vi "ExecuteState.vi"(0 "StateIn":T7 {"ILoad" format="%_6g"; "Fault Registers" format="%016x"; "VLoad" format="%_6g"; "VDCLink" format="%_6g"; "Detected Frequency" format="%1_6g"}, 1 "Interfaces":T2, 7 "methods":T1, 9 "params":refnum<class "JSON Null.lvclass">, 11 "error in (no error)":errorcluster) -> (4 "StateOut":T7 {"ILoad" format="%_6g"; "Fault Registers" format="%016x"; "VLoad" format="%_6g"; "VDCLink" format="%_6g"; "Detected Frequency" format="%1_6g"}, 15 "error out":errorcluster)   [LabVIEW 2017, in "AppStateMachine runtime.lvclass"]
uses:
  AppStateMachine runtime.lvclass
  State.ctl
  StateId.ctl
  LED_Color.ctl
  Interfaces.ctl
  <vilib>/NI/NI JSONRPC Server Framework/Classes/Server/JSONRPC Server.lvclass
  <instrlib>/_niInstr/Instruction Framework/v1/Host/Instruction Target/niInstr Instruction Target v1 Host.lvclass
  <instrlib>/_niInstr/Instruction Framework/v1/Host/Instruction Framework Context/niInstr Instruction Framework Context v1 Host.lvclass
  FPGA/FPGAtypedef.ctl
  <vilib>/NI/PowerElectronicsControl/ThreePhasePLL/Interface/InterfaceRef.ctl
  <vilib>/NI/PowerElectronicsControl/ActiveFrontEnd/AFE_Interface/InterfaceRef.ctl
  <vilib>/NI/PowerElectronicsControl/Buck-Boost/RealTime/Interface.ctl
  Support/methods.ctl
  <vilib>/NI/JSON Support for LabVIEW/JSON Data Classes/JSON Datatype/JSON Null.lvclass
  <vilib>/rvi/Analysis/control/PID/Typedef/niFpgaPID_PIGains.ctl
  <vilib>/rvi/Analysis/control/PID/Typedef/niFpgaPID_OutputRange.ctl
  <vilib>/NI/PowerElectronicsControl/ActiveFrontEnd/AFE/PI_Settings.ctl
  <vilib>/NI/PowerElectronicsControl/Buck-Boost/RealTime/TuningParameters.ctl
  <vilib>/NI/PowerElectronicsControl/Buck-Boost/FPGA/contState.ctl
  <vilib>/NI/JSON Support for LabVIEW/JSON Data Classes/JSON Object/JSON Object.lvclass
  C:/Program Files (x86)/National Instruments/LabVIEW 2017/vi.lib/NI/JSON Support for LabVIEW/JSON Data Classes/JSON Datatype/JSON Null.lvclass
  <vilib>/NI/JSON Support for LabVIEW/JSON Data Classes/JSON Helper/To More Specific Type (Object).vi
  <vilib>/NI/JSON Support for LabVIEW/JSON Data Classes/JSON Object/Get Value (Object).vi
  <vilib>/Utility/error.llb/Error Cluster From Error Code.vi
  <vilib>/rvi/errors/niLvFpgaAdjustHostInterfaceError.vi
  <vilib>/NI/JSON Support for LabVIEW/JSON Data Classes/JSON Helper/To More Specific Type (Numeric).vi
  <vilib>/NI/JSON Support for LabVIEW/JSON Data Classes/JSON Numeric/Read value (Numeric).vi
  <vilib>/rvi/interface/nirviReadWriteControl/nirviReadWriteControl.xnode
  <vilib>/NI/PowerElectronicsControl/ThreePhasePLL/Interface/ThreePhasePLLInterface.lvlib
  <vilib>/NI/JSON Support for LabVIEW/JSON Data Classes/JSON Helper/JSON Helper.lvclass
  <vilib>/NI/PowerElectronicsControl/ActiveFrontEnd/AFE_Interface/AFE_interface.lvlib
  <vilib>/NI/PowerElectronicsControl/ActiveFrontEnd/AFE/ActiveFrontEnd.lvlib
  <vilib>/NI/PowerElectronicsControl/Buck-Boost/RealTime/BuckBoostInterface.lvlib
  <vilib>/NI/PowerElectronicsControl/Buck-Boost/FPGA/BuckBoost.lvlib
  NiFpgaLv.dll
  <vilib>/rvi/interface/Simulation/niFpgaSimulationCallBeginRW.vi
  <vilib>/NI/JSON Support for LabVIEW/JSON Data Classes/JSON Basic Type/JSON Literal.lvclass
  <vilib>/NI/JSON Support for LabVIEW/JSON Data Classes/JSON Numeric/JSON Numeric.lvclass
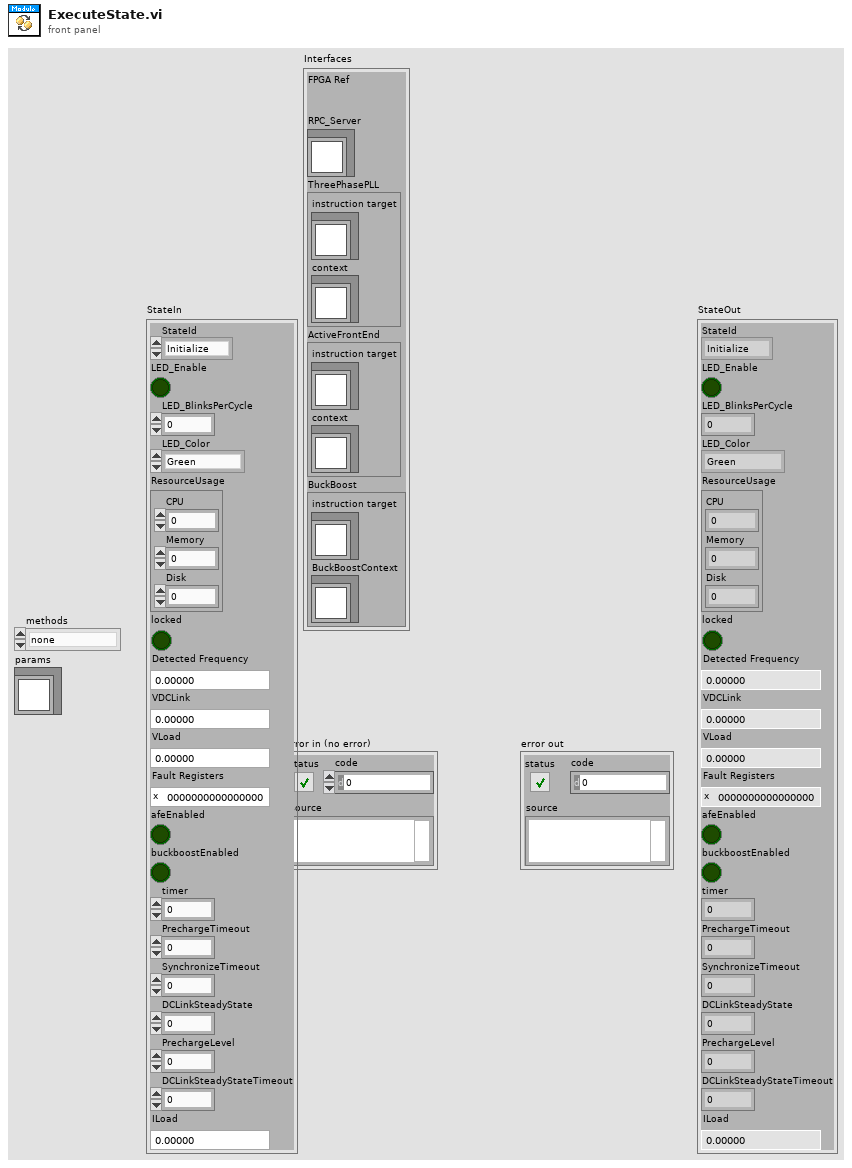
[diagram p1: front panel]
types:
  T1 = typedef "AppStateMachine runtime.lvclass/methods.ctl" = enum16{"none", "echo", "GetResourceUsage", "CheckConnection", "CurrentState", "GoToSafeState", "ClearSafeState", "AvailableLogs", "ForceLogTrigger", "GoToTuneAFE", "GoToTunePLL", "GoToTuneBuckBoost", "TurnOnSystem", "TurnOffSystem", "PrechargeSystem", "SetPLL_Tune", "SetBuckBoostSetpoint", "SetAFE_tune", "SetBuckBoostTune", "CompleteTuning", "PllSettings", "AfeSettings", "BuckBoostSettings", "enableAfe", "disableAfe", "enableBuckBoost", "disableBuckBoost"}
  T2 = typedef "AppStateMachine runtime.lvclass/Interfaces.ctl" = cluster{"FPGA Ref":T3, "RPC_Server":refnum<class "JSONRPC Server.lvclass">, "ThreePhasePLL":T4, "ActiveFrontEnd":T5, "BuckBoost":T6}
  T3 = typedef "AppStateMachine runtime.lvclass/FPGAtypedef.ctl" = refnum<k20>
  T4 = typedef "ThreePhasePLLInterface.lvlib/InterfaceRef.ctl" = cluster{"instruction target":refnum<class "niInstr Instruction Target v1 Host.lvclass">, "context":refnum<class "niInstr Instruction Framework Context v1 Host.lvclass">}
  T5 = typedef "AFE_interface.lvlib/InterfaceRef.ctl" = cluster{"instruction target":refnum<class "niInstr Instruction Target v1 Host.lvclass">, "context":refnum<class "niInstr Instruction Framework Context v1 Host.lvclass">}
  T6 = typedef "BuckBoostInterface.lvlib/Interface.ctl" = cluster{"instruction target":refnum<class "niInstr Instruction Target v1 Host.lvclass">, "BuckBoostContext":refnum<class "niInstr Instruction Framework Context v1 Host.lvclass">}
  T7 = typedef "AppStateMachine runtime.lvclass/State.ctl" = cluster{"StateId":T8, "LED_Enable":bool, "LED_BlinksPerCycle":i32, "LED_Color":T9, "ResourceUsage":cluster{"CPU":dbl, "Memory":dbl, "Disk":dbl}, "locked":bool, "Detected Frequency":dbl, "VDCLink":dbl, "VLoad":dbl, "Fault Registers":u64, "afeEnabled":bool, "buckboostEnabled":bool, "timer":u32, "PrechargeTimeout":u32, "SynchronizeTimeout":u32, "DCLinkSteadyState":dbl, "PrechargeLevel":dbl, "DCLinkSteadyStateTimeout":u32, "ILoad":dbl}
  T8 = typedef "AppStateMachine runtime.lvclass/StateId.ctl" = enum16{"Initialize", "Idle", "TunePLL", "TuneAFE", "TuneBuckBoost", "Precharge", "Synchronize", "Ready", "EnableAFE", "EnableBuckBoost", "Powered", "SafeState", "UnrecoverableSafeState"}
  T9 = typedef "AppStateMachine runtime.lvclass/LED_Color.ctl" = enum16{"Green", "Yellow"}
  T10 = typedef "BuckBoost.lvlib/contState.ctl" = enum16{"disabled", "manual", "normal", "perturb"}
  T11 = typedef "niFpgaPID_OutputRange.ctl" = cluster{"output high (Inf)":sgl, "output low (-Inf)":sgl}
  T12 = typedef "niFpgaPID_PIGains.ctl" = cluster{"proportional gain":sgl, "integral gain":sgl}
  T13 = typedef "ActiveFrontEnd.lvlib/PI_Settings.ctl" = cluster{"gains":T12, "output range":T11, "PI_state":enum8{"idle", "normal", "manual", "perturbance"}, "reset":bool, "manual":sgl}
  T14 = typedef "BuckBoostInterface.lvlib/TuningParameters.ctl" = cluster{"gains":T12, "manualInput":sgl, "rampRate":sgl, "pertAmp":sgl, "pertFreq":sgl, "controlFreq":sgl, "state":T10}
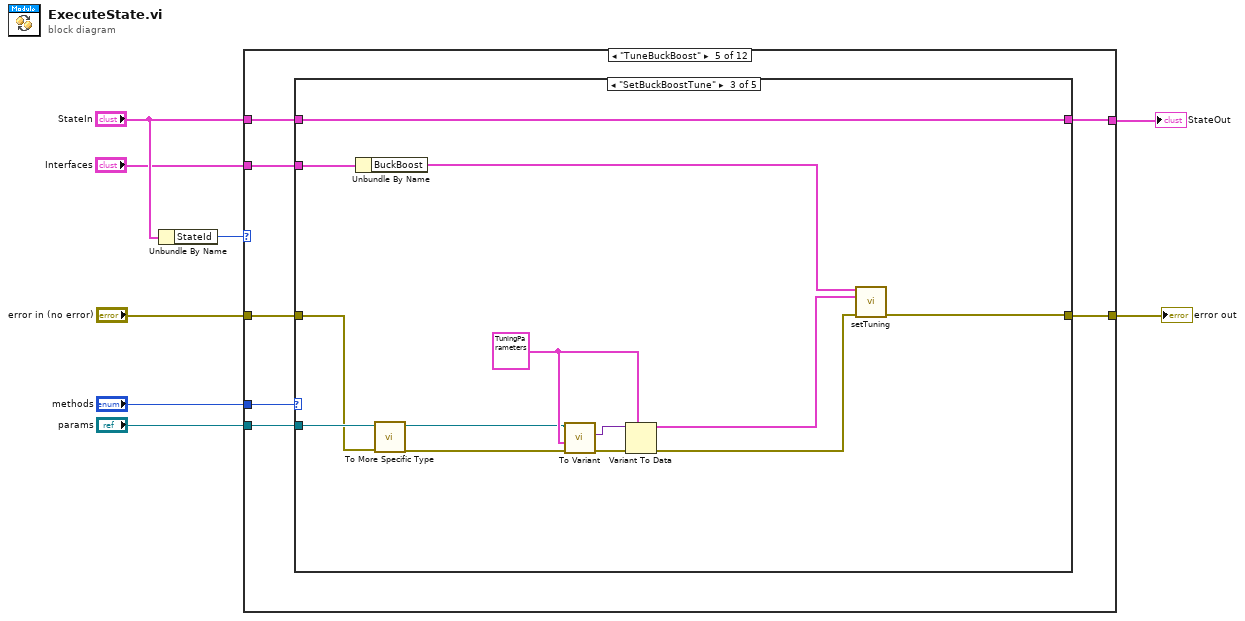
[diagram p0: block diagram]
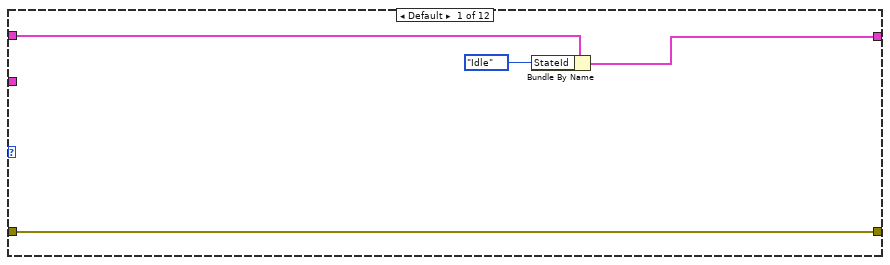
[diagram p2: hidden frame]
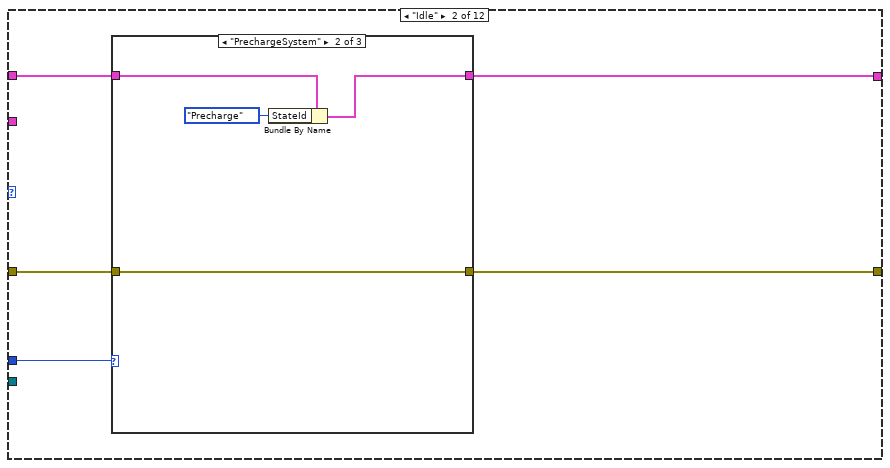
[diagram p3: hidden frame]
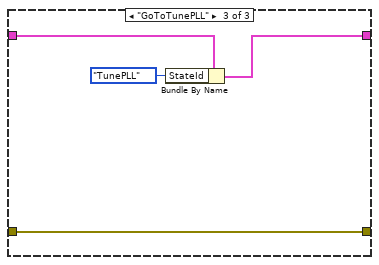
[diagram p5: hidden frame]
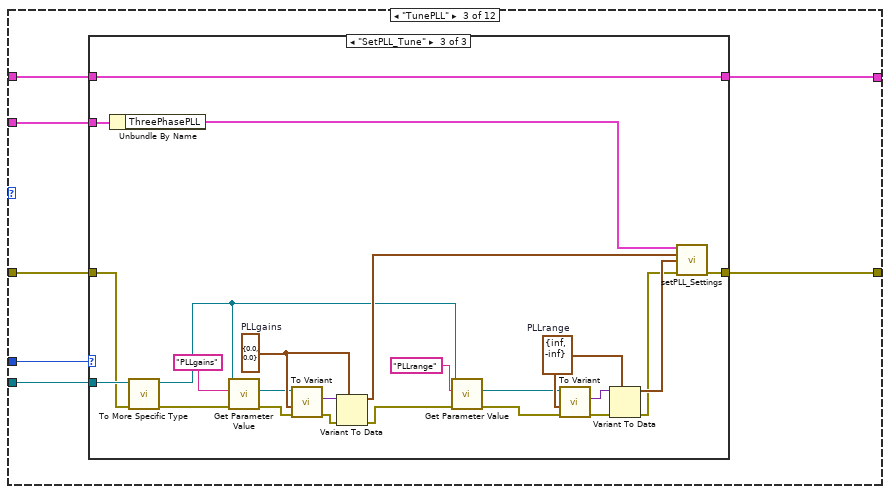
[diagram p6: hidden frame]
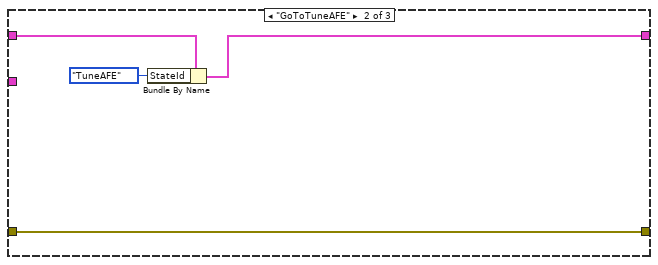
[diagram p8: hidden frame]
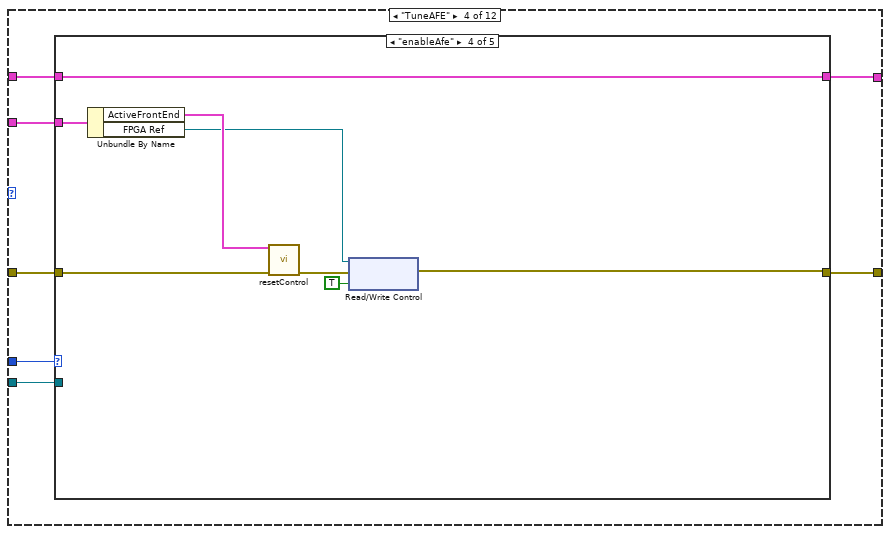
[diagram p9: hidden frame]
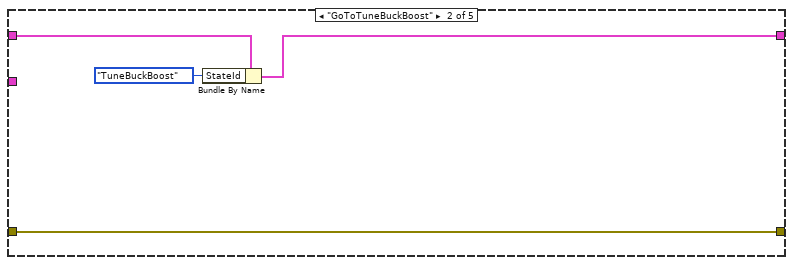
[diagram p11: hidden frame]
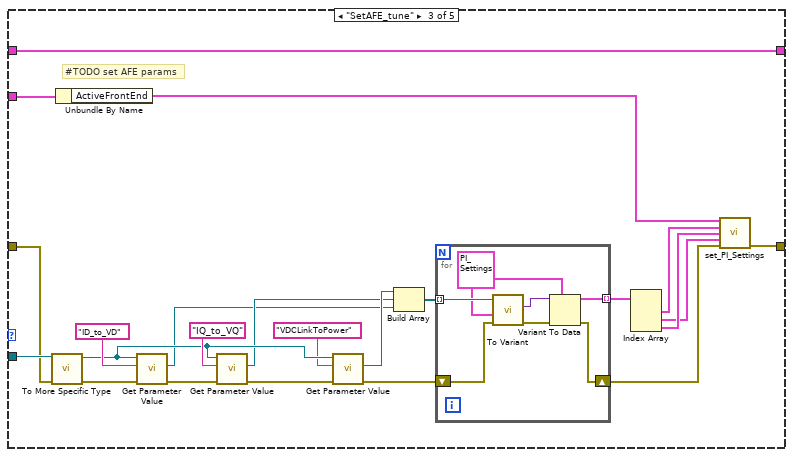
[diagram p12: hidden frame]
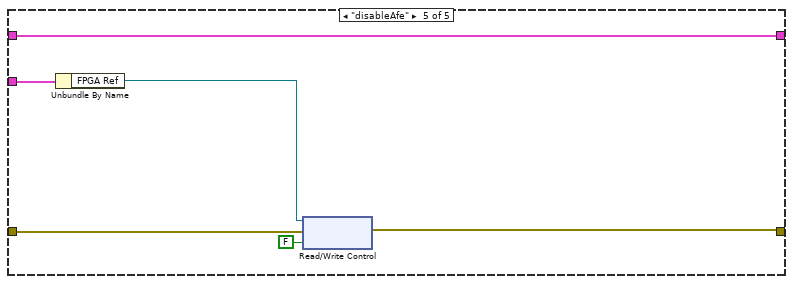
[diagram p13: hidden frame]
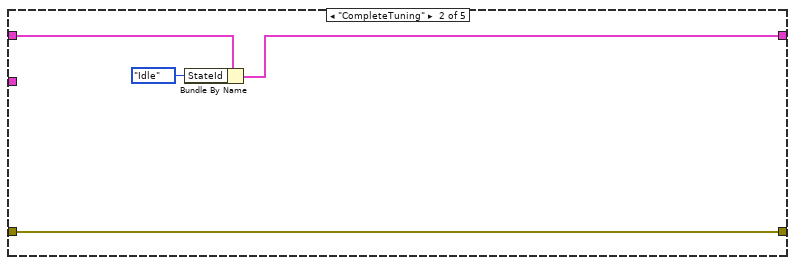
[diagram p15: hidden frame]
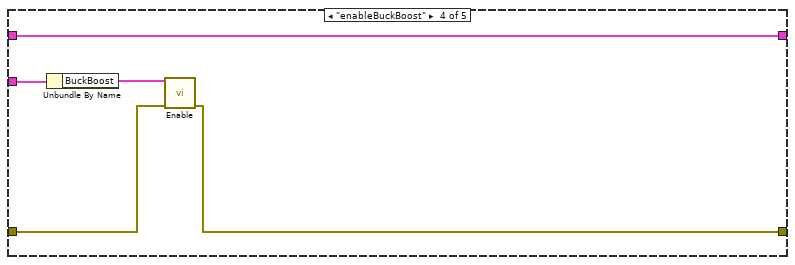
[diagram p16: hidden frame]
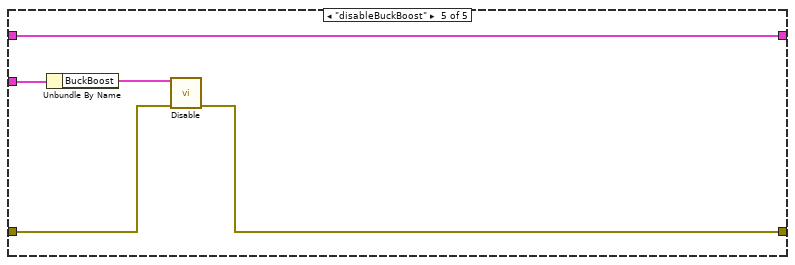
[diagram p17: hidden frame]
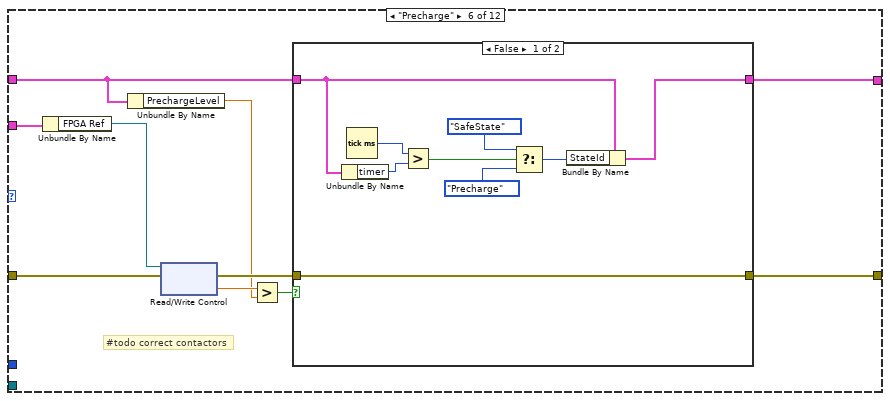
[diagram p18: hidden frame]
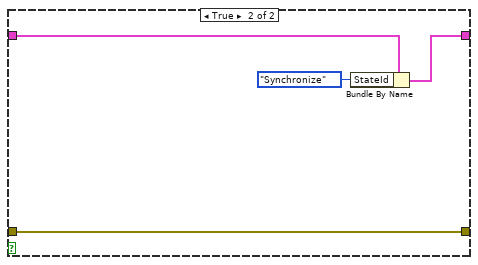
[diagram p19: hidden frame]
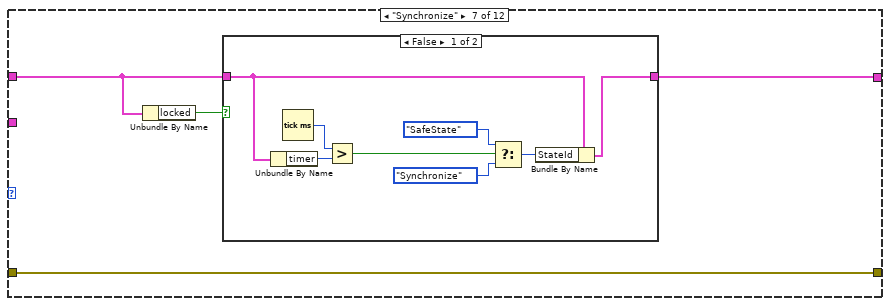
[diagram p20: hidden frame]
diagram:
  n1 = Unbundle By Name("StateIn") -> ("StateId"=w3:T8)
  n2 = case shown="\"TuneBuckBoost\"" w3 {
    tunnel: "error in (no error)" -> [w12 w14 w31 w68 w125 w165 w184 w197 w220 w240 w248 w272]
    tunnel: [w12 w13 w30 w67 w124 w160 w184 w196 w220 w232 w247 w269] -> w8
    tunnel: "params" -> [_ _ w29 w66 w123 _ _ _ _ _ w245 _]
    tunnel: "methods" -> [_ w17 w34 w71 w128 _ _ w198 _ _ w249 w273]
    tunnel: "Interfaces" -> [_ _ w28 w65 w122 w166 _ _ _ w241 w246 _]
    tunnel: "StateIn" -> [w11 w16 w33 w70 w127 w159 w182 w200 w212 w244 w251 w271]
    tunnel: [w9 w15 w32 w69 w126 w167 w183 w199 w211 w243 w250 w270] -> w6
    frame Default {
      n3 = Bundle By Name(cluster=w11, "StateId"=StateId."Idle") -> (w9:T7)
    }
    frame "Idle" {
      n4 = case shown="\"PrechargeSystem\"" w17 {
        tunnel: w16 -> [w19 w23 w27]
        tunnel: [w19 w21 w25] -> w15
        tunnel: w14 -> [w18 w20 w24]
        tunnel: [w18 w20 w24] -> w13
        frame "none", Default {
        }
        frame "PrechargeSystem" {
          n5 = Bundle By Name(cluster=w23, "StateId"=StateId."Precharge") -> (w21:T7)
        }
        frame "GoToTunePLL" {
          n6 = Bundle By Name(cluster=w27, "StateId"=StateId."TunePLL") -> (w25:T7)
        }
      }
    }
    frame "TunePLL" {
      n7 = case shown="\"SetPLL_Tune\"" w34 {
        tunnel: w33 -> [w36 w39 w64]
        tunnel: [w36 w38 w64] -> w32
        tunnel: w31 -> [w35 w37 w59]
        tunnel: [w35 w37 w62] -> w30
        tunnel: w29 -> [_ _ w60]
        tunnel: w28 -> [_ _ w63]
        frame "none", Default {
        }
        frame "GoToTuneAFE" {
          n8 = Bundle By Name(cluster=w39, "StateId"=StateId."TuneAFE") -> (w38:T7)
        }
        frame "SetPLL_Tune" {
          w55 = T11 {"output high (Inf)"=inf, "output low (-Inf)"=-inf}  # PLLrange
          w57 = T12 {"proportional gain"=0.0, "integral gain"=0.0}  # PLLgains
          n9 = Unbundle By Name(w63) -> ("ThreePhasePLL"=w61:T4)
          n10 = call-poly <vilib>:"To More Specific Type.vi"("error in (no error)"=w59, "JSON Datatype in"=w60) -> ("error out"=w46:errorcluster, "JSON Datatype out"=w48:refnum<class "JSON Object.lvclass">)  [unwired: 8 in]
          n11 = call-poly <vilib>:"Get Parameter Value.vi"("error in (no error)"=w46, "key"="PLLgains", "JSON Object in"=w48) -> ("error out"=w45:errorcluster, "value"=w49:refnum<class "JSON Object.lvclass">)  [unwired: 7 in]
          n12 = call <vilib>:"To Variant.vi"("error in (no error)"=w45, "datatype and defaults"=w57, "JSON Datatype in"=w49) -> ("error out"=w44:errorcluster, "Variant"=w58:variant)  [unwired: 6 in, 1 out]
          n13 = Variant To Data(error in=w44, type=w57, Variant=w58) -> (data=w54:T12, error out=w42:errorcluster)
          n14 = call-poly <vilib>:"Get Parameter Value.vi"("error in (no error)"=w42, "key"="PLLrange", "JSON Object in"=w48) -> ("error out"=w41:errorcluster, "value"=w43:refnum<class "JSON Object.lvclass">)  [unwired: 7 in]
          n15 = call <vilib>:"To Variant.vi"("error in (no error)"=w41, "datatype and defaults"=w55, "JSON Datatype in"=w43) -> ("error out"=w52:errorcluster, "Variant"=w56:variant)  [unwired: 6 in, 1 out]
          n16 = Variant To Data(error in=w52, type=w55, Variant=w56) -> (data=w53:T11, error out=w51:errorcluster)
          n17 = call <vilib>:"setPLL_Settings.vi"("Interface in"=w61, "PLLgains"=w54, "PLLrange"=w53, "error in"=w51) -> ("error out"=w62:errorcluster)  [unwired: 10 in, 1 out]
        }
      }
    }
    frame "TuneAFE" {
      n18 = case shown="\"enableAfe\"" w71 {
        tunnel: w70 -> [w73 w76 w100 w115 w121]
        tunnel: [w73 w75 w100 w115 w121] -> w69
        tunnel: w68 -> [w72 w74 w98 w114 w116]
        tunnel: [w72 w74 w93 w108 w117] -> w67
        tunnel: w66 -> [_ _ w99 _ _]
        tunnel: w65 -> [_ _ w95 w113 w120]
        frame "none", Default {
        }
        frame "GoToTuneBuckBoost" {
          n19 = Bundle By Name(cluster=w76, "StateId"=StateId."TuneBuckBoost") -> (w75:T7)
        }
        frame "SetAFE_tune" {
          # "#TODO set AFE params"
          n20 = call-poly <vilib>:"To More Specific Type.vi"("error in (no error)"=w98, "JSON Datatype in"=w99) -> ("error out"=w97:errorcluster, "JSON Datatype out"=w90:refnum<class "JSON Object.lvclass">)  [unwired: 8 in]
          n21 = Unbundle By Name(w95) -> ("ActiveFrontEnd"=w94:T5)
          n22 = call-poly <vilib>:"Get Parameter Value.vi"("error in (no error)"=w97, "key"="ID_to_VD", "JSON Object in"=w90) -> ("error out"=w92:errorcluster, "value"=w85:refnum<class "JSON Object.lvclass">)  [unwired: 7 in]
          n23 = call-poly <vilib>:"Get Parameter Value.vi"("error in (no error)"=w92, "key"="IQ_to_VQ", "JSON Object in"=w90) -> ("error out"=w88:errorcluster, "value"=w86:refnum<class "JSON Object.lvclass">)  [unwired: 7 in]
          n24 = call-poly <vilib>:"Get Parameter Value.vi"("error in (no error)"=w88, "key"="VDCLinkToPower", "JSON Object in"=w90) -> ("error out"=w83:errorcluster, "value"=w87:refnum<class "JSON Object.lvclass">)  [unwired: 7 in]
          n25 = Build Array(w87, w86, w85) -> (w84:refnum<class "JSON Object.lvclass">[])
          n26 = for {
            tunnel: w84 -> [w107] mode=indexing
            shift-right: [w101] -> w82
            shift-left: w83 -> [w106]
            tunnel: [w102] -> w81 mode=indexing
            w103 = T13 {"gains"={"proportional gain"=0.0, "integral gain"=0.0}, "output range"={"output high (Inf)"=inf, "output low (-Inf)"=-inf}, "PI_state"=enum."idle", "reset"=FALSE, "manual"=0.0} ("ID_to_VD")
            n27 = call <vilib>:"To Variant.vi"("error in (no error)"=w106, "datatype and defaults"=w103, "JSON Datatype in"=w107) -> ("error out"=w105:errorcluster, "Variant"=w104:variant)  [unwired: 6 in, 1 out]
            n28 = Variant To Data(error in=w105, type=w103, Variant=w104) -> (data=w102:T13, error out=w101:errorcluster)
          }
          n29 = Index Array(array=w81) -> (element #1=w80:T13, element #2=w78:T13, element #3=w79:T13)  [unwired: 3 in]
          n30 = call <vilib>:"set_PI_Settings.vi"("Interface in"=w94, "VDCLinkToPower"=w80, "ID_to_VD"=w79, "IQ_to_VQ"=w78, "error in"=w82) -> ("error out"=w93:errorcluster)  [unwired: 9 in, 1 out]
        }
        frame "enableAfe" {
          n31 = Unbundle By Name(w113) -> ("ActiveFrontEnd"=w112:T5, "FPGA Ref"=w110:T3)
          n32 = call <vilib>:"resetControl.vi"("Interface in"=w112, "error in"=w114) -> ("error out"=w111:errorcluster)  [unwired: 12 in, 1 out]
          n33 = xnode "Read/Write Control"("FPGA VI Reference In"=w110, "error in"=w111, "enableAFE"=TRUE) -> ("error out"=w108:errorcluster)  [unwired: 1 out]
        }
        frame "disableAfe" {
          n34 = Unbundle By Name(w120) -> ("FPGA Ref"=w119:T3)
          n35 = xnode "Read/Write Control"("FPGA VI Reference In"=w119, "error in"=w116, "enableAFE"=FALSE) -> ("error out"=w117:errorcluster)  [unwired: 1 out]
        }
      }
    }
    frame "TuneBuckBoost" {
      n36 = case shown="\"SetBuckBoostTune\"" w128 {
        tunnel: w127 -> [w130 w133 w147 w148 w153]
        tunnel: [w130 w132 w147 w148 w153] -> w126
        tunnel: w125 -> [w129 w131 w142 w150 w156]
        tunnel: [w129 w131 w140 w149 w154] -> w124
        tunnel: w123 -> [_ _ w145 _ _]
        tunnel: w122 -> [_ _ w146 w152 w157]
        frame "none", Default {
        }
        frame "CompleteTuning" {
          n37 = Bundle By Name(cluster=w133, "StateId"=StateId."Idle") -> (w132:T7)
        }
        frame "SetBuckBoostTune" {
          w138 = T14 {"gains"={"proportional gain"=0.0, "integral gain"=0.0}, "manualInput"=0.0, "rampRate"=0.0, "pertAmp"=0.0, "pertFreq"=0.0, "controlFreq"=0.0, "state"=enum."disabled"} ("TuningParameters")
          n38 = Unbundle By Name(w146) -> ("BuckBoost"=w141:T6)
          n39 = call-poly <vilib>:"To More Specific Type.vi"("error in (no error)"=w142, "JSON Datatype in"=w145) -> ("error out"=w135:errorcluster, "JSON Datatype out"=w136:refnum<class "JSON Object.lvclass">)  [unwired: 8 in]
          n40 = call <vilib>:"To Variant.vi"("error in (no error)"=w135, "datatype and defaults"=w138, "JSON Datatype in"=w136) -> ("error out"=w144:errorcluster, "Variant"=w143:variant)  [unwired: 6 in, 1 out]
          n41 = Variant To Data(error in=w144, type=w138, Variant=w143) -> (data=w137:T14, error out=w139:errorcluster)
          n42 = call <vilib>:"setTuning.vi"("Interface in"=w141, "TuningParameters"=w137, "error in (no error)"=w139) -> ("error out"=w140:errorcluster)  [unwired: 11 in, 1 out]
        }
        frame "enableBuckBoost" {
          n43 = Unbundle By Name(w152) -> ("BuckBoost"=w151:T6)
          n44 = call <vilib>:"Enable.vi"("Interface in"=w151, "error in (no error)"=w150) -> ("error out"=w149:errorcluster)  [unwired: 12 in, 1 out]
        }
        frame "disableBuckBoost" {
          n45 = Unbundle By Name(w157) -> ("BuckBoost"=w155:T6)
          n46 = call <vilib>:"Disable.vi"("Interface in"=w155, "error in (no error)"=w156) -> ("error out"=w154:errorcluster)  [unwired: 12 in, 1 out]
        }
      }
    }
    frame "Precharge" {
      # "#todo correct contactors"
      n47 = Unbundle By Name(w166) -> ("FPGA Ref"=w164:T3)
      n48 = Unbundle By Name(w159) -> ("PrechargeLevel"=w158:dbl)
      n49 = xnode "Read/Write Control"("FPGA VI Reference In"=w164, "error in"=w165) -> ("error out"=w161:errorcluster, "VDCLink"=w163:sgl)  [unwired: 1 out]
      n50 = Greater?(x=w163, y=w158) -> (0:w162:bool)
      n51 = case shown="False" w162 {
        tunnel: [w169 w179] -> w167
        tunnel: w159 -> [w174 w178]
        tunnel: w161 -> [w168 w177]
        tunnel: [w168 w177] -> w160
        frame False {
          n52 = Unbundle By Name(w174) -> ("timer"=w176:u32)
          n53 = Tick Count (ms)() -> (millisecond timer value=w175:u32)
          n54 = Greater?(x=w175, y=w176) -> (0:w171:bool)
          n55 = Select(t=StateId."SafeState" ("StateId"), s=w171, f=StateId."Precharge" ("StateId")) -> (s? t:f=w170:T8)
          n56 = Bundle By Name(cluster=w174, "StateId"=w170) -> (w169:T7)
        }
        frame True {
          n57 = Bundle By Name(cluster=w178, "StateId"=StateId."Synchronize") -> (w179:T7)
        }
      }
    }
    frame "Synchronize" {
      n58 = Unbundle By Name(w182) -> ("locked"=w181:bool)
      n59 = case shown="False" w181 {
        tunnel: [w185 w195] -> w183
        tunnel: w182 -> [w186 w193]
        frame False {
          n60 = Unbundle By Name(w186) -> ("timer"=w192:u32)
          n61 = Tick Count (ms)() -> (millisecond timer value=w191:u32)
          n62 = Greater?(x=w191, y=w192) -> (0:w190:bool)
          n63 = Select(t=StateId."SafeState" ("StateId"), s=w190, f=StateId."Synchronize" ("StateId")) -> (s? t:f=w189:T8)
          n64 = Bundle By Name(cluster=w186, "StateId"=w189) -> (w185:T7)
        }
        frame True {
          n65 = Bundle By Name(cluster=w193, "StateId"=StateId."Ready") -> (w195:T7)
        }
      }
    }
    frame "Ready" {
      n66 = case shown="\"TurnOnSystem\"" w198 {
        tunnel: w200 -> [w202 w205 w209]
        tunnel: [w202 w204 w208] -> w199
        tunnel: w197 -> [w201 w203 w207]
        tunnel: [w201 w203 w207] -> w196
        frame "none", Default {
        }
        frame "TurnOnSystem" {
          n67 = Bundle By Name(cluster=w205, "StateId"=StateId."EnableAFE") -> (w204:T7)
        }
        frame "TurnOffSystem" {
          n68 = Bundle By Name(cluster=w209, "StateId"=StateId."Idle") -> (w208:T7)
        }
      }
    }
    frame "EnableAFE" {
      n69 = Unbundle By Name(w212) -> ("DCLinkSteadyState"=w217:dbl, "VDCLink"=w214:dbl)
      n70 = Multiply(x=w217, y=0.9) -> (x*y=w215:dbl)
      n71 = Multiply(x=w217, y=1.1 ("x")) -> (x*y=w219:dbl)
      n72 = In Range and Coerce(upper limit=w219, x=w214, lower limit=w215) -> (In Range?=w213:bool)  [unwired: 1 out]
      n73 = case shown="True" w213 {
        tunnel: w212 -> [w225 w230]
        tunnel: [w224 w229] -> w211
        frame False {
          n74 = Tick Count (ms)() -> (millisecond timer value=w227:u32)
          n75 = Unbundle By Name(w225) -> ("timer"=w228:u32)
          n76 = Greater?(x=w227, y=w228) -> (0:w226:bool)
          n77 = Select(t=StateId."SafeState" ("StateId"), s=w226, f=StateId."EnableAFE") -> (s? t:f=w222:T8)
          n78 = Bundle By Name(cluster=w225, "StateId"=w222) -> (w224:T7)
        }
        frame True {
          n79 = Bundle By Name(cluster=w230, "StateId"=StateId."EnableBuckBoost") -> (w229:T7)
        }
      }
    }
    frame "EnableBuckBoost" {
      n80 = Unbundle By Name(w241) -> ("BuckBoost"=w236:T6, "FPGA Ref"=w239:T3)
      n81 = xnode "Read/Write Control"("FPGA VI Reference In"=w239, "error in"=w240, "I_setpt"=sgl 0.0) -> ("error out"=w237:errorcluster)  [unwired: 1 out]
      n82 = call <vilib>:"reset.vi"("Interface in"=w236, "error in (no error)"=w237) -> ("Interface out"=w234:T6, "error out"=w235:errorcluster)  [unwired: 12 in]
      n83 = call <vilib>:"setState.vi"("Interface in"=w234, "state"=contState."normal", "error in (no error)"=w235) -> ("error out"=w232:errorcluster)  [unwired: 11 in, 1 out]
      n84 = Bundle By Name(cluster=w244, "StateId"=StateId."Powered") -> (w243:T7)
    }
    frame "Powered" {
      n85 = case shown="\"SetBuckBoostSetpoint\"" w249 {
        tunnel: w251 -> [w253 w257 w268]
        tunnel: [w253 w256 w268] -> w250
        tunnel: w248 -> [w252 w254 w263]
        tunnel: [w252 w254 w266] -> w247
        tunnel: w246 -> [_ _ w267]
        tunnel: w245 -> [_ _ w264]
        frame "none", Default {
        }
        frame "TurnOffSystem" {
          n86 = Bundle By Name(cluster=w257, "StateId"=StateId."Idle") -> (w256:T7)
        }
        frame "SetBuckBoostSetpoint" {
          n87 = Unbundle By Name(w267) -> ("FPGA Ref"=w265:T3)
          n88 = call-poly <vilib>:"To More Specific Type.vi"("error in (no error)"=w263, "JSON Datatype in"=w264) -> ("error out"=w262:errorcluster, "JSON Numeric out"=w261:refnum<class "JSON Numeric.lvclass">)  [unwired: 8 in]
          n89 = call-poly <vilib>:"Read Value.vi"("error in (no error)"=w262, "default value"=0.0, "JSON Numeric in"=w261) -> ("error out"=w259:errorcluster, "value"=w258:dbl)  [unwired: 7 in]
          n90 = xnode "Read/Write Control"("FPGA VI Reference In"=w265, "error in"=w259, "I_setpt"=w258) -> ("error out"=w266:errorcluster)  [unwired: 1 out]
        }
      }
    }
    frame "SafeState" {
      n91 = case shown="\"ClearSafeState\"" w273 {
        tunnel: w272 -> [w277 w278]
        tunnel: w271 -> [w275 w281]
        tunnel: [w274 w279] -> w270
        tunnel: [w277 w278] -> w269
        frame Default {
          n92 = Bundle By Name(cluster=w275, "StateId"=StateId."SafeState") -> (w274:T7)
        }
        frame "ClearSafeState" {
          n93 = Bundle By Name(cluster=w281, "StateId"=StateId."Idle") -> (w279:T7)
        }
      }
    }
  }
  "error out" <- w8
  "StateOut" <- w6
